vi "Generate_SDA_SCL.vi"(0 "Data":T2={"Vmin"=0.0, "Vmax"=1.0, "Input"="", "Off_Set (uS)"=0.0, "T_HD_STA (uS)"=0.0, "Sample_Per_Us"=0.0, "T_HD_DAT (uS)"=0.0, "T_SU_DAT (uS)"=0.0, "Frequency (kHz)"=0.0, "T_SU_STO"=0.0, "T_Off (uS)"=0.0, "T_On (uS)"=0.0, "T_BUF"=0.0, "Target_Address"=0, "Selected_Register_Address"=0, "Byte_Array"=[], "Target_Name"="", "Register_Name"=[], "Register_Address"=[], "Ring"=0} {"Target_Type" items=["Select Item", ""]; "Selected_Register_Address" format="%x"; "Target_Address" format="%x"}, 7 "Data_Sequence":T1[](array[typedef])=[enum."Start", enum."Byte", enum."Ack_Nack", enum."Byte", enum."Stop"], 11 "Error_In":errorcluster) -> (4 "Waveform Graph":waveform(dbl)[](graph)=[{"t0"=timestamp(0 s since 1904-01-01), "dt"=1e-09, "Y"=array[98005 elements]}, {"t0"=timestamp(0 s since 1904-01-01), "dt"=1e-09, "Y"=array[98005 elements]}], 15 "Error_Out":errorcluster)   [LabVIEW 2023]
doc: "Core Protocol generator which generates the analog waveform that represents the data given."
uses:
  Controls/Converted_Data.ctl
  Controls/Menu_Ring.ctl
  Controls/I2C_States.ctl
  Controls/Control 6.ctl
  Controls/Byte_Generator_Data.ctl
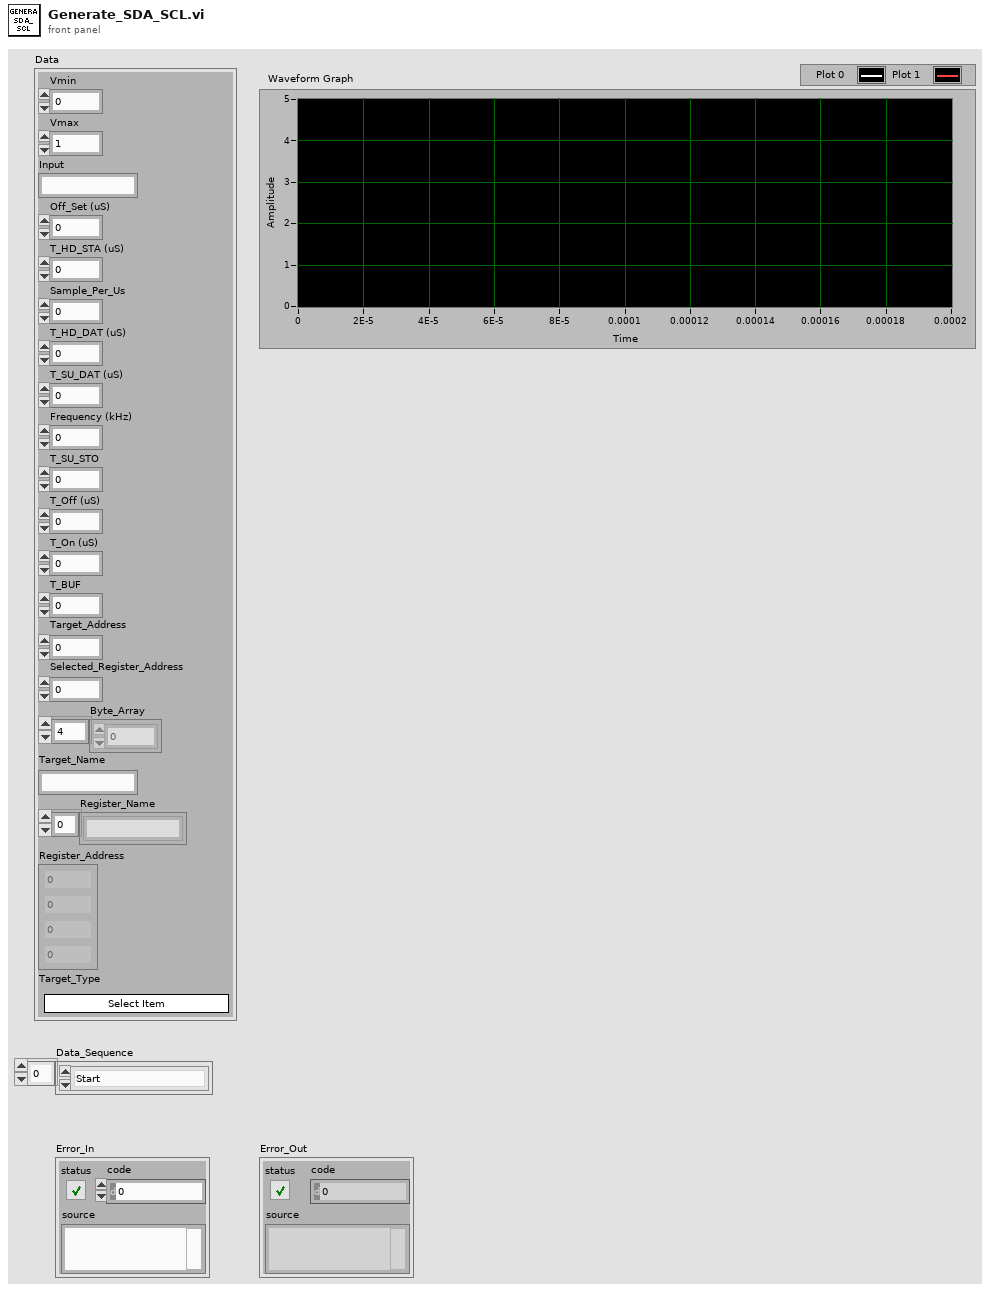
[diagram p1: front panel]
types:
  T1 = typedef "I2C_States.ctl" = enum16{"Start", "Byte", "Ack_Nack", "Stop"}
  T2 = typedef "Converted_Data.ctl" = cluster{"Vmin":dbl, "Vmax":dbl, "Input":string, "Off_Set (uS)":dbl, "T_HD_STA (uS)":dbl, "Sample_Per_Us":dbl, "T_HD_DAT (uS)":dbl, "T_SU_DAT (uS)":dbl, "Frequency (kHz)":dbl, "T_SU_STO":dbl, "T_Off (uS)":dbl, "T_On (uS)":dbl, "T_BUF":dbl, "Target_Address":u16, "Selected_Register_Address":u8, "Byte_Array":u8[], "Target_Name":string, "Register_Name":string[], "Register_Address":u8[], "Ring":T3}
  T3 = typedef "Menu_Ring.ctl" = u16
  T4 = typedef "Control 6.ctl" = cluster{"SCL":dbl[], "SDA":dbl[]}
  T5 = typedef "Byte_Generator_Data.ctl" = cluster{"SDA":dbl[], "SCL":dbl[], "Previous_Bit":dbl, "Initial_SCL_Bit":bool, "Data_Hold_Time":i32, "Data_Time":i32, "T_On":i32, "T_Off":i32, "Vmin":dbl, "Vmax":dbl}
  T6 = typedef "Time_Parameter.ctl" = cluster{"Vmin":dbl, "Vmax":dbl, "Off_Set (uS)":i32, "T_HD_STA (uS)":i32, "Sample_Per_Us":i32, "T_HD_DAT (uS)":i32, "T_SU_DAT (uS)":i32, "Data_Time (uS)":i32, "T_SU_STO":i32, "T_Off (uS)":i32, "T_On (uS)":i32, "T_BUF":i32, "Byte_Array":u8[]}
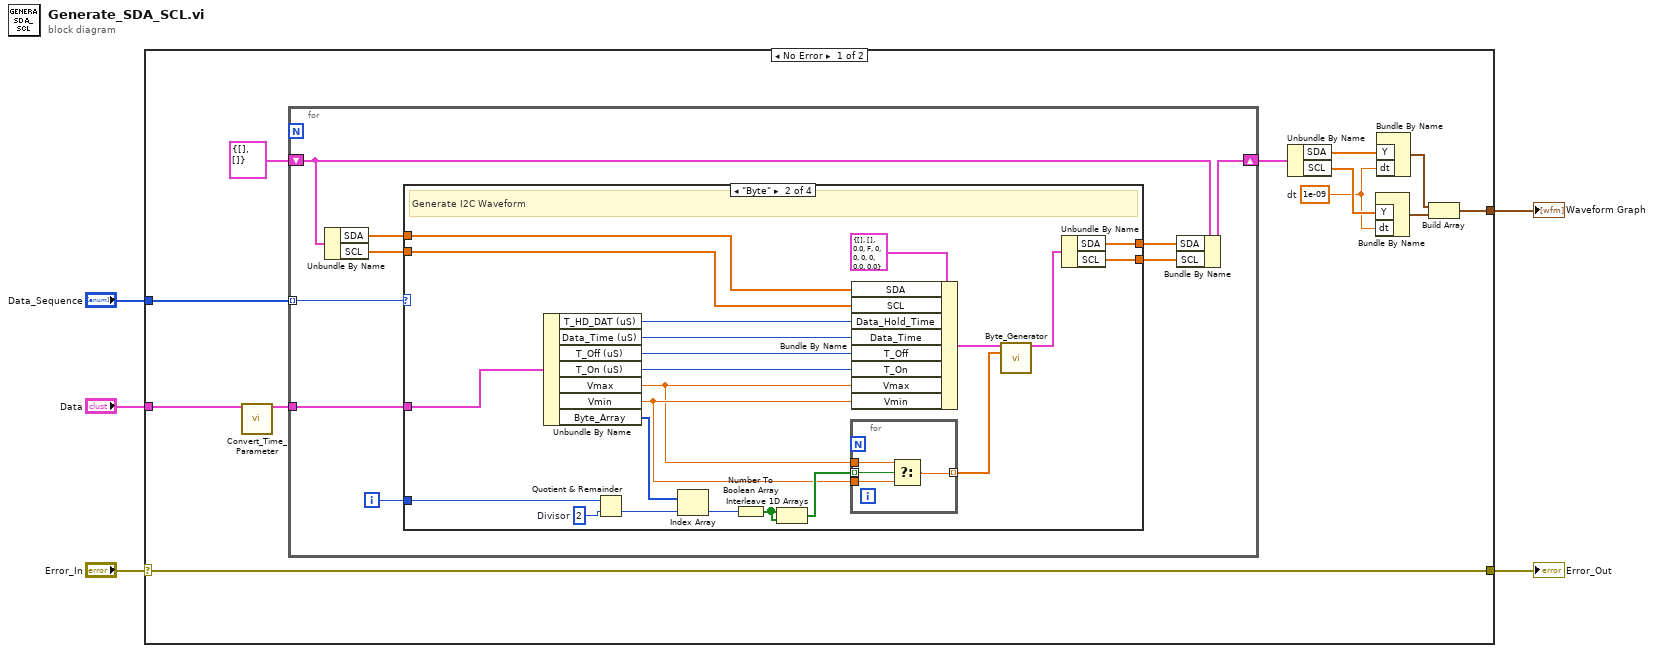
[diagram p0: block diagram]
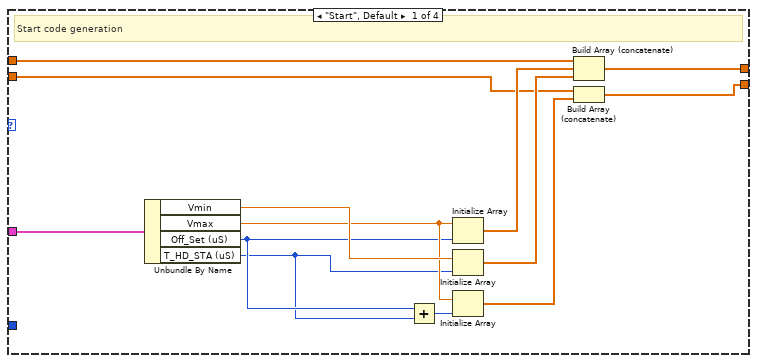
[diagram p2: hidden frame]
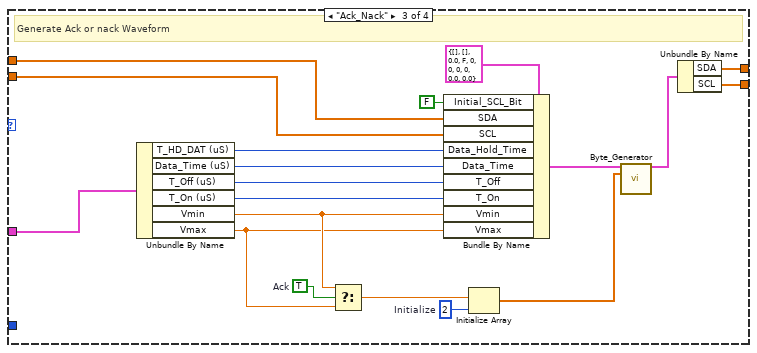
[diagram p3: hidden frame]
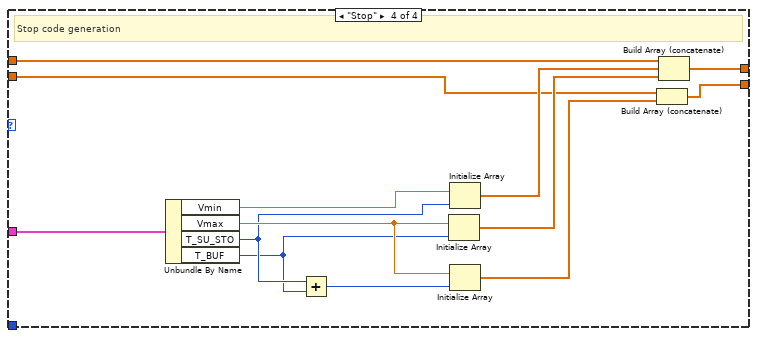
[diagram p4: hidden frame]
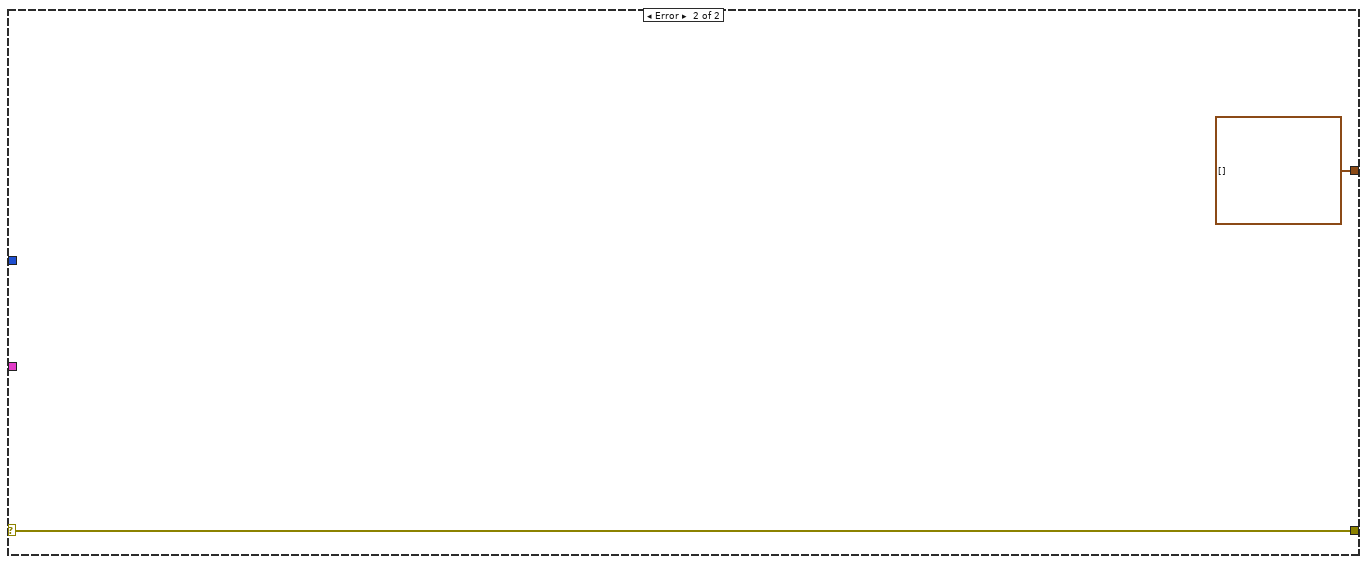
[diagram p5: hidden frame]
diagram:
  n1 = case shown="No Error" "Error_In" {
    selector: "Error_In" -> [w6 w99]
    tunnel: "Data" -> [w17 _]
    tunnel: "Data_Sequence" -> [w16 _]
    tunnel: [w12 waveform(dbl)[] []] -> w3
    tunnel: [w6 w99] -> w1
    frame No Error {
      w7 = 1e-09  # dt
      n2 = call "Convert_Time_Parameter.vi"("Data"=w17) -> ("Converted_Data"=w15:T6)  [unwired: 14 in]
      n3 = for {
        tunnel: w16 -> [w26] mode=indexing
        tunnel: w15 -> [w25]
        shift-right: [w21] -> w10
        shift-left: T4 {"SCL"=[], "SDA"=[]} -> [w22]
        i -> [w18]
        n4 = Unbundle By Name(w22) -> ("SDA"=w24:dbl[], "SCL"=w23:dbl[])
        n5 = case shown="\"Byte\"" w26 {
          tunnel: w25 -> [w38 w57 w81 w97]
          tunnel: w24 -> [w34 w53 w69 w93]
          tunnel: w23 -> [w32 w52 w76 w92]
          tunnel: [w33 w51 w75 w90] -> w19
          tunnel: [w30 w50 w74 w89] -> w20
          tunnel: w18 -> [_ w49 _ _]
          frame "Start", Default {
            # "Start code generation"
            n6 = Unbundle By Name(w38) -> ("Vmin"=w37:dbl, "Vmax"=w36:dbl, "Off_Set (uS)"=w28:i32, "T_HD_STA (uS)"=w27:i32)
            n7 = Add(x=w28, y=w27) -> (x+y=w29:i32)
            n8 = Initialize Array(w36, w28) -> (w39:dbl[])
            n9 = Initialize Array(w37, w27) -> (w35:dbl[])
            n10 = Initialize Array(w36, w29) -> (w31:dbl[])
            n11 = Build Array (concatenate)(w34, w39, w35) -> (w33:dbl[])
            n12 = Build Array (concatenate)(w32, w31) -> (w30:dbl[])
          }
          frame "Byte" {
            w48 = 2  # Divisor
            # "Generate I2C Waveform"
            n13 = Unbundle By Name(w57) -> ("T_HD_DAT (uS)"=w54:i32, "Data_Time (uS)"=w45:i32, "T_Off (uS)"=w55:i32, "T_On (uS)"=w56:i32, "Vmax"=w40:dbl, "Vmin"=w41:dbl, "Byte_Array"=w42:u8[])
            n14 = Quotient & Remainder(x=w49, y=w48) -> (floor(x/y)=w47:i32)  [unwired: 1 out]
            n15 = Index Array(array=w42, index=w47) -> (element=w46:u8)
            n16 = Number To Boolean Array(number=w46) -> (Boolean array=w61:bool[])
            n17 = Interleave 1D Arrays(w61, w61) -> (w44:bool[])
            n18 = for {
              tunnel: w41 -> [w65]
              tunnel: w44 -> [w64] mode=indexing
              tunnel: [w63] -> w43 mode=indexing
              tunnel: w40 -> [w62]
              n19 = Select(t=w62, s=w64, f=w65) -> (s? t:f=w63:dbl)
            }
            n20 = Bundle By Name(cluster=T5 {"SDA"=[], "SCL"=[], "Previous_Bit"=0.0, "Initial_SCL_Bit"=FALSE, "Data_Hold_Time"=0, "Data_Time"=0, "T_On"=0, "T_Off"=0, "Vmin"=0.0, "Vmax"=0.0}, "SDA"=w53, "SCL"=w52, "Data_Hold_Time"=w54, "Data_Time"=w45, "T_Off"=w55, "T_On"=w56, "Vmax"=w40, "Vmin"=w41) -> (w59:T5)
            n21 = call "Byte_Generator.vi"("Data_In"=w59, "Byte_Array"=w43) -> ("Data_Out"=w58:T5)  [unwired: 13 in]
            n22 = Unbundle By Name(w58) -> ("SDA"=w51:dbl[], "SCL"=w50:dbl[])
          }
          frame "Ack_Nack" {
            w70 = TRUE  # Ack
            w73 = 2  # Initialize
            # "Generate Ack or nack Waveform"
            n23 = Unbundle By Name(w81) -> ("T_HD_DAT (uS)"=w78:i32, "Data_Time (uS)"=w77:i32, "T_Off (uS)"=w79:i32, "T_On (uS)"=w80:i32, "Vmin"=w67:dbl, "Vmax"=w66:dbl)
            n24 = Select(t=w67, s=w70, f=w66) -> (s? t:f=w71:dbl)
            n25 = Bundle By Name(cluster=T5 {"SDA"=[], "SCL"=[], "Previous_Bit"=0.0, "Initial_SCL_Bit"=FALSE, "Data_Hold_Time"=0, "Data_Time"=0, "T_On"=0, "T_Off"=0, "Vmin"=0.0, "Vmax"=0.0}, "Initial_SCL_Bit"=FALSE, "SDA"=w69, "SCL"=w76, "Data_Hold_Time"=w78, "Data_Time"=w77, "T_Off"=w79, "T_On"=w80, "Vmin"=w67, "Vmax"=w66) -> (w83:T5)
            n26 = Initialize Array(w71, w73) -> (w72:dbl[])
            n27 = call "Byte_Generator.vi"("Data_In"=w83, "Byte_Array"=w72) -> ("Data_Out"=w82:T5)  [unwired: 13 in]
            n28 = Unbundle By Name(w82) -> ("SDA"=w75:dbl[], "SCL"=w74:dbl[])
          }
          frame "Stop" {
            # "Stop code generation"
            n29 = Unbundle By Name(w97) -> ("Vmin"=w87:dbl, "Vmax"=w88:dbl, "T_SU_STO"=w86:i32, "T_BUF"=w85:i32)
            n30 = Add(x=w86, y=w85) -> (x+y=w91:i32)
            n31 = Initialize Array(w88, w85) -> (w96:dbl[])
            n32 = Initialize Array(w87, w86) -> (w95:dbl[])
            n33 = Initialize Array(w88, w91) -> (w94:dbl[])
            n34 = Build Array (concatenate)(w92, w94) -> (w89:dbl[])
            n35 = Build Array (concatenate)(w93, w95, w96) -> (w90:dbl[])
          }
        }
        n36 = Bundle By Name(cluster=w22, "SDA"=w19, "SCL"=w20) -> (w21:T4)
      }
      n37 = Unbundle By Name(w10) -> ("SDA"=w9:dbl[], "SCL"=w8:dbl[])
      n38 = Bundle By Name("Y"=w8, "dt"=w7) -> (w11:waveform(dbl))  [unwired: 1 in]
      n39 = Bundle By Name("Y"=w9, "dt"=w7) -> (w13:waveform(dbl))  [unwired: 1 in]
      n40 = Build Array(w13, w11) -> (w12:waveform(dbl)[])
    }
    frame Error {
    }
  }
  "Waveform Graph" <- w3
  "Error_Out" <- w1
